vi "CMC_Homework_03.vi"() -> ()   [LabVIEW 2013]
panel:
  in  "stop":bool
  out "Middle Bound":dbl
  in  "Lower Bound":dbl
  in  "Upper Bound":dbl
  in  "Tolerance":dbl min=0.0
  out "Calculated Tolerance":dbl
  out "Roots of F(x) found to Tolerance":string[](array[string])
  # "Created in Collaboration with Sarah Bailey & Alex Offredi"
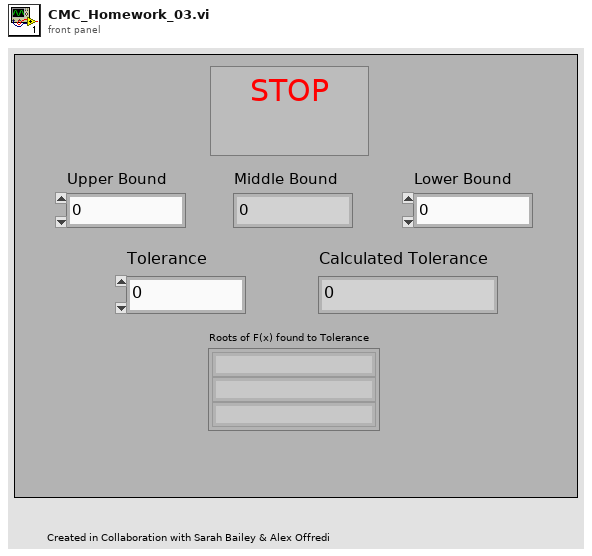
[diagram p1: front panel]
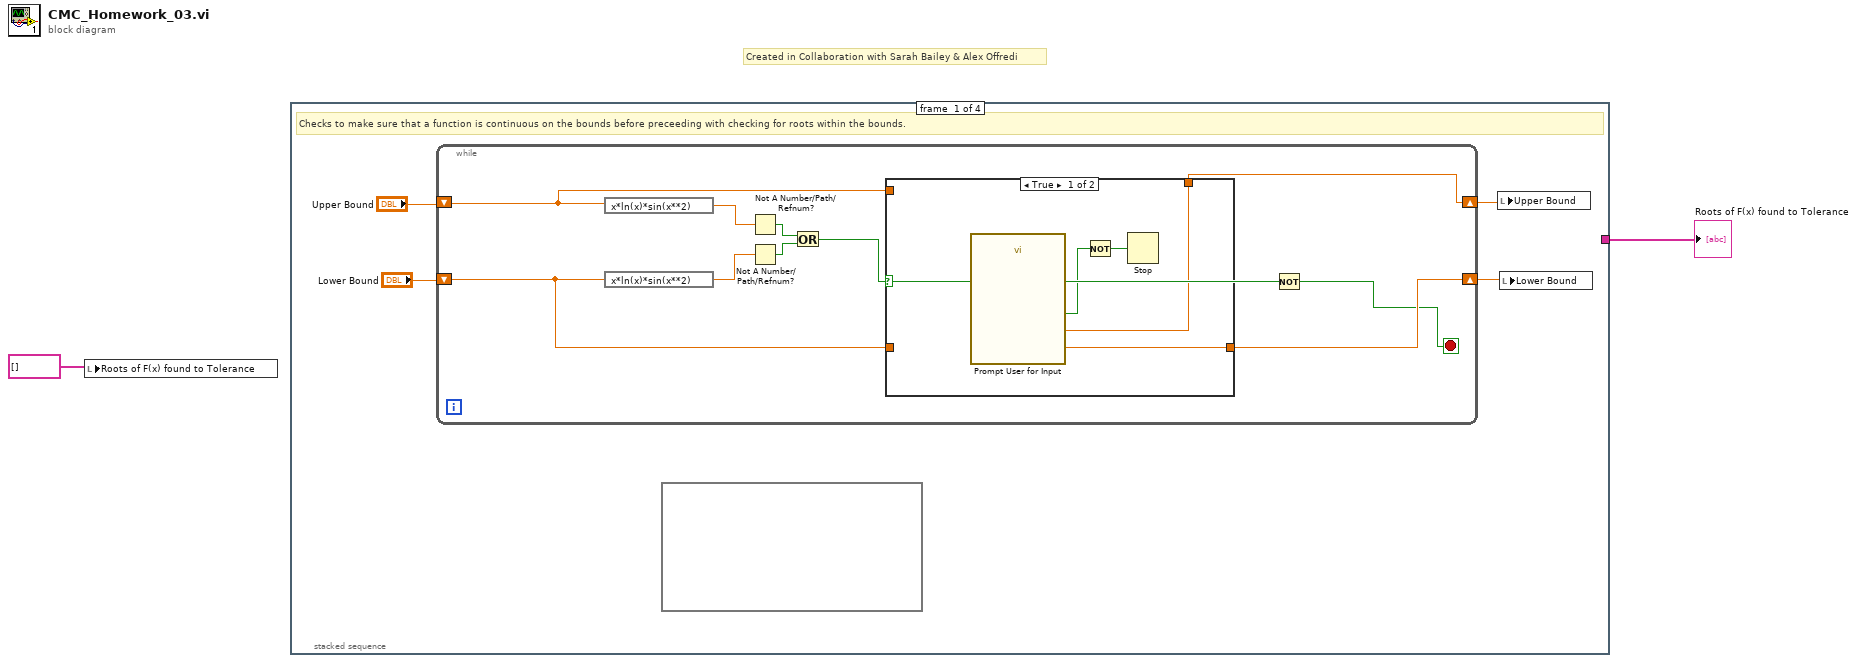
[diagram p0: block diagram]
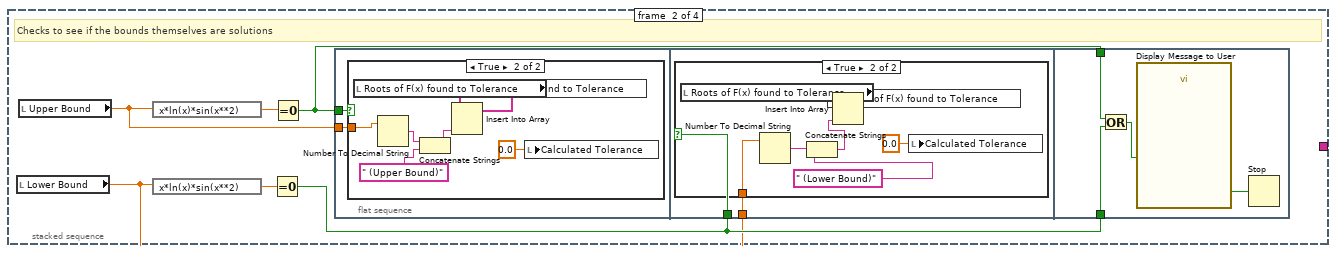
[diagram p3: hidden frame]
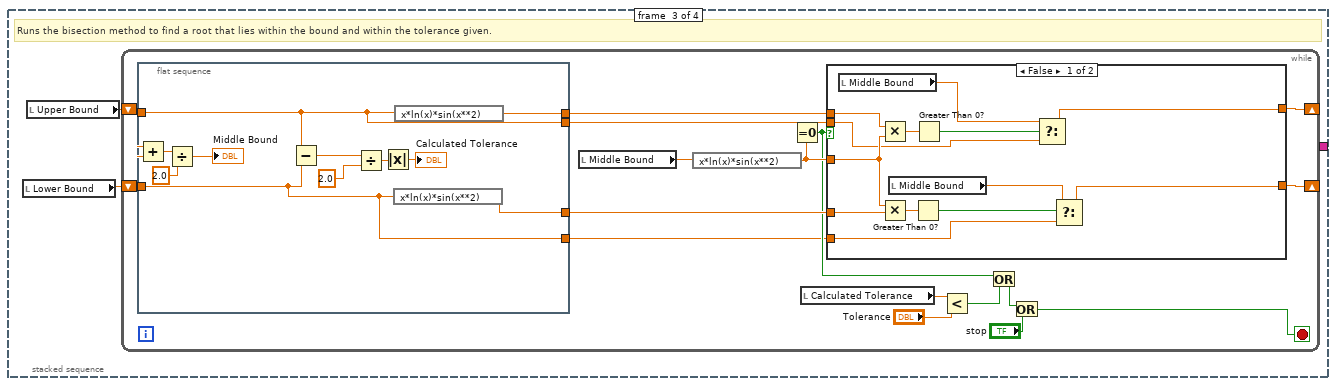
[diagram p6: hidden frame]
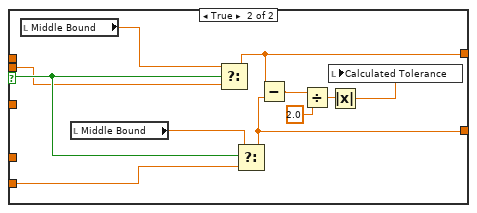
[diagram p7: hidden frame]
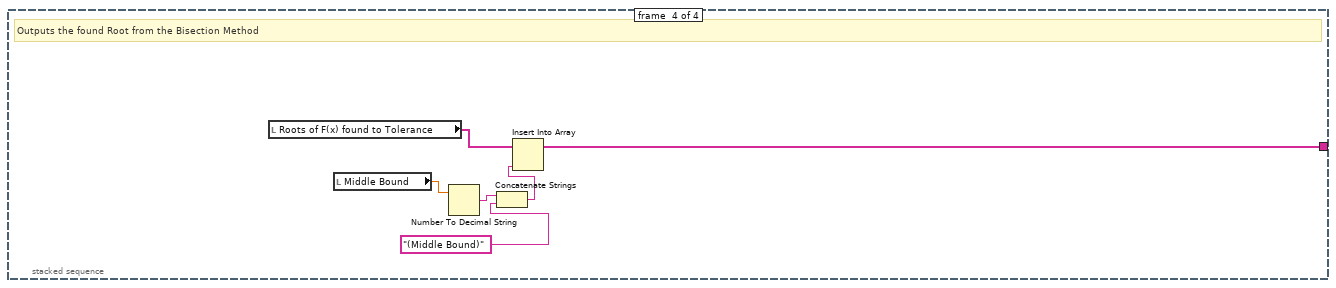
[diagram p8: hidden frame]
diagram:
  # "Created in Collaboration with Sarah Bailey & Alex Offredi"
  n1 = local write "Roots of F(x) found to Tolerance"(string[] [] ("Roots of F(x) found to Tolerance")) -> ()
  n2 = stacked-sequence {
    tunnel: [_ _ _ w105] -> w2
    frame #0 {
      # "Checks to make sure that a function is continuous on the bounds before preceeding with checking for roots within the bounds."
      n3 = while {
        shift-right: [w12] -> w3
        shift-left: "Upper Bound" -> [w9]
        shift-right: [w11] -> w4
        shift-left: "Lower Bound" -> [w8]
        stop <- w7 stop-if-true
        n4 = expression code="x*ln(x)*sin(x**2)"(w9) -> (w15:dbl)
        n5 = expression code="x*ln(x)*sin(x**2)"(w8) -> (w16:dbl)
        n6 = Not A Number/Path/Refnum?(number/path/refnum=w15) -> (NaN/Path/Refnum?=w13:bool)
        n7 = Not A Number/Path/Refnum?(number/path/refnum=w16) -> (NaN/Path/Refnum?=w14:bool)
        n8 = Or(x=w13, y=w14) -> (x .or. y?=w10:bool)
        n9 = case shown="True" w10 {
          tunnel: [w18 w21] -> w12
          tunnel: [w17 w22] -> w11
          tunnel: w9 -> [_ w21]
          tunnel: w8 -> [_ w22]
          frame True {
            n10 = call "Prompt User for Input"() -> ("Lower Bound"=w17:dbl, "Upper Bound"=w18:dbl, "OK"=w19:bool)  [unwired: 16 in, 1 out]
            n11 = Not(x=w19) -> (.not. x?=w20:bool)
            n12 = Stop(stop? (T)=w20) -> ()
          }
          frame False {
          }
        }
        n13 = Not(x=w10) -> (.not. x?=w7:bool)
      }
      n14 = formula code=""() -> ()
      n15 = local write "Upper Bound"(w3) -> ()
      n16 = local write "Lower Bound"(w4) -> ()
    }
    frame #1 {
      # "Checks to see if the bounds themselves are solutions"
      n17 = local read "Lower Bound"() -> (w23:dbl)
      n18 = local read "Upper Bound"() -> (w24:dbl)
      n19 = expression code="x*ln(x)*sin(x**2)"(w24) -> (w28:dbl)
      n20 = expression code="x*ln(x)*sin(x**2)"(w23) -> (w27:dbl)
      n21 = Equal To 0?(x=w27) -> (x = 0?=w26:bool)
      n22 = Equal To 0?(x=w28) -> (x = 0?=w25:bool)
      n23 = flat-sequence {
        tunnel: w25 -> [w30]
        tunnel: w24 -> [w29]
        tunnel: w26 -> [w38]
        tunnel: w23 -> [w39]
        tunnel: w26 -> [w49]
        tunnel: w25 -> [w50]
        frame #0 {
          n24 = case shown="True" w30 {
            tunnel: w29 -> [_ w35]
            frame False {
            }
            frame True {
              n25 = local read "Roots of F(x) found to Tolerance"() -> (w37:string[])
              n26 = Number To Decimal String(number=w35) -> (decimal integer string=w34:string)  [unwired: 1 in]
              n27 = Concatenate Strings(w34, " (Upper Bound)") -> (w32:string)
              n28 = Insert Into Array(array=w37, new element=w32) -> (w36:string[])  [unwired: 1 in]
              n29 = local write "Roots of F(x) found to Tolerance"(w36) -> ()
              n30 = local write "Calculated Tolerance"(0.0 ("Calculated Tolerance")) -> ()
            }
          }
        }
        frame #1 {
          n31 = case shown="True" w38 {
            tunnel: w39 -> [_ w44]
            frame False {
            }
            frame True {
              n32 = local read "Roots of F(x) found to Tolerance"() -> (w46:string[])
              n33 = Number To Decimal String(number=w44) -> (decimal integer string=w43:string)  [unwired: 1 in]
              n34 = Concatenate Strings(w43, " (Lower Bound)") -> (w41:string)
              n35 = Insert Into Array(array=w46, new element=w41) -> (w45:string[])  [unwired: 1 in]
              n36 = local write "Roots of F(x) found to Tolerance"(w45) -> ()
              n37 = local write "Calculated Tolerance"(0.0 ("Calculated Tolerance")) -> ()
            }
          }
        }
        frame #2 {
          n38 = Or(x=w50, y=w49) -> (x .or. y?=w48:bool)
          n39 = call "Display Message to User"("Enable"=w48) -> ("OK"=w47:bool)  [unwired: 9 in, 1 out]
          n40 = Stop(stop? (T)=w47) -> ()
        }
      }
    }
    frame #2 {
      # "Runs the bisection method to find a root that lies within the bound and within the tolerance given."
      n41 = local read "Lower Bound"() -> (w51:dbl)
      n42 = local read "Upper Bound"() -> (w52:dbl)
      n43 = while {
        shift-right: [w64] -> _
        shift-left: w52 -> [w69]
        shift-right: [w63] -> _
        shift-left: w51 -> [w68]
        stop <- w60 stop-if-true
        n44 = flat-sequence {
          tunnel: w69 -> [w95]
          tunnel: w68 -> [w94]
          tunnel: [w99] -> w66
          tunnel: [w98] -> w65
          tunnel: [w95] -> w54
          tunnel: [w94] -> w53
          frame #0 {
            n45 = Add(x=w95, y=w94) -> (x+y=w103:dbl)
            n46 = Divide(x=w103, y=2.0) -> (x/y=→"Middle Bound":dbl)
            n47 = Subtract(x=w95, y=w94) -> (x-y=w101:dbl)
            n48 = Divide(x=w101, y=2.0) -> (x/y=w97:dbl)
            n49 = Absolute Value(x=w97) -> (abs(x)=→"Calculated Tolerance":dbl)
            n50 = expression code="x*ln(x)*sin(x**2)"(w94) -> (w98:dbl)
            n51 = expression code="x*ln(x)*sin(x**2)"(w95) -> (w99:dbl)
          }
        }
        n52 = local read "Middle Bound"() -> (w67:dbl)
        n53 = expression code="x*ln(x)*sin(x**2)"(w67) -> (w58:dbl)
        n54 = Equal To 0?(x=w58) -> (x = 0?=w57:bool)
        n55 = local read "Calculated Tolerance"() -> (w61:dbl)
        n56 = case shown="False" w57 {
          selector: w57 -> [_ w85]
          tunnel: w66 -> [w72 _]
          tunnel: w65 -> [w74 _]
          tunnel: [w79 w89] -> w64
          tunnel: w58 -> [w73 _]
          tunnel: [w76 w88] -> w63
          tunnel: w54 -> [w71 w83]
          tunnel: w53 -> [w70 w84]
          frame False {
            n57 = local read "Middle Bound"() -> (w75:dbl)
            n58 = Multiply(x=w72, y=w73) -> (x*y=w82:dbl)
            n59 = Multiply(x=w73, y=w74) -> (x*y=w81:dbl)
            n60 = local read "Middle Bound"() -> (w77:dbl)
            n61 = Greater Than 0?(x=w81) -> (x > 0?=w78:bool)
            n62 = Greater Than 0?(x=w82) -> (x > 0?=w80:bool)
            n63 = Select(t=w75, s=w80, f=w71) -> (s? t:f=w79:dbl)
            n64 = Select(t=w77, s=w78, f=w70) -> (s? t:f=w76:dbl)
          }
          frame True {
            n65 = local read "Middle Bound"() -> (w92:dbl)
            n66 = local read "Middle Bound"() -> (w93:dbl)
            n67 = Select(t=w92, s=w85, f=w83) -> (s? t:f=w89:dbl)
            n68 = Select(t=w93, s=w85, f=w84) -> (s? t:f=w88:dbl)
            n69 = Subtract(x=w89, y=w88) -> (x-y=w90:dbl)
            n70 = Divide(x=w90, y=2.0) -> (x/y=w87:dbl)
            n71 = Absolute Value(x=w87) -> (abs(x)=w86:dbl)
            n72 = local write "Calculated Tolerance"(w86) -> ()
          }
        }
        n73 = Less?(x=w61, y="Tolerance") -> (x < y?=w56:bool)
        n74 = Or(x=w57, y=w56) -> (x .or. y?=w55:bool)
        n75 = Or(x=w55, y="stop") -> (x .or. y?=w60:bool)
      }
    }
    frame #3 {
      # "Outputs the found Root from the Bisection Method"
      n76 = local read "Roots of F(x) found to Tolerance"() -> (w110:string[])
      n77 = local read "Middle Bound"() -> (w109:dbl)
      n78 = Number To Decimal String(number=w109) -> (decimal integer string=w108:string)  [unwired: 1 in]
      n79 = Concatenate Strings(w108, "(Middle Bound)") -> (w106:string)
      n80 = Insert Into Array(array=w110, new element=w106) -> (w105:string[])  [unwired: 1 in]
    }
  }
  "Roots of F(x) found to Tolerance" <- w2
